vi "Drivers Folder.vi"(3 "Relative Path (\"\" - Folder)":string) -> (1 "Drivers Folder":path)   [LabVIEW 2011]
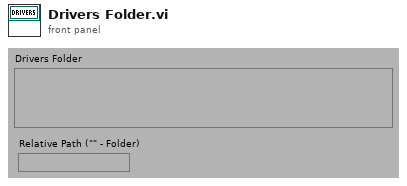
[diagram p1: front panel]
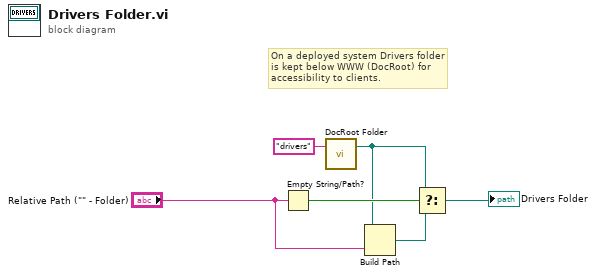
[diagram p0: block diagram]
diagram:
  # "On a deployed system Drivers folder\nis kept below WWW (DocRoot) for\naccessibility to clients."
  n1 = Empty String/Path?(string/path="Relative Path (\"\" - Folder)") -> (empty?=w5:bool)
  n2 = call "DocRoot Folder.vi"("Relative Path (\"\" - Folder)"="drivers" ("name or relative path")) -> ("DocumentRoot Folder"=w2:path)  [unwired: 2 in]
  n3 = Build Path(base path=w2, name or relative path="Relative Path (\"\" - Folder)") -> (appended path=w3:path)
  n4 = Select(t=w2, s=w5, f=w3) -> (s? t:f=→"Drivers Folder":path)
